vi "CircleShape.vi"(1 "Precision":i32, 2 "Y initial":dbl format="%#_13g", 3 "X initial":dbl format="%#_13g", 4 "Radius":dbl format="%#_13g") -> (0 "Output Point":dbl[][](array[numeric]))   [LabVIEW 2013]
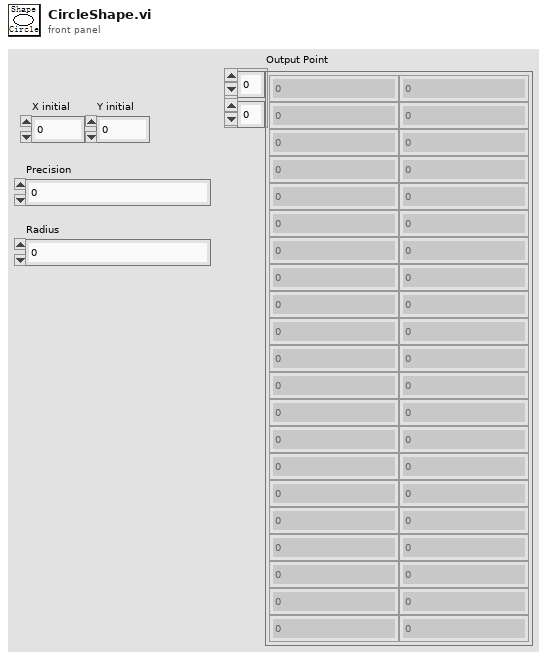
[diagram p1: front panel]
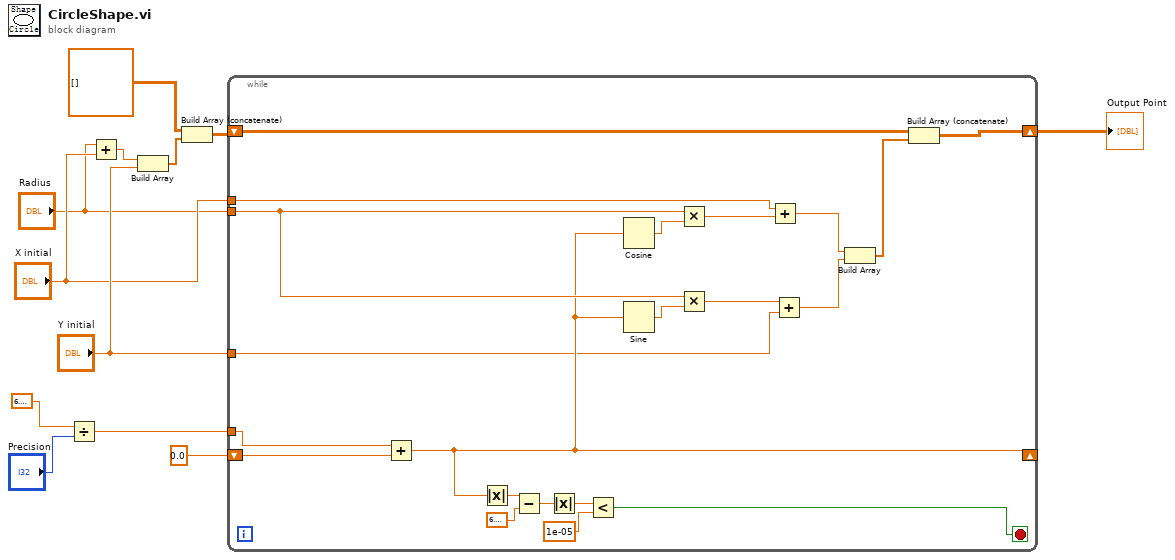
[diagram p0: block diagram]
diagram:
  n1 = Divide(x=6.283185307179586, y="Precision") -> (x/y=w9:dbl)
  n2 = Add(x="Radius", y="X initial") -> (x+y=w3:dbl)
  n3 = Build Array(w3, "Y initial") -> (w4:dbl[])
  n4 = Build Array (concatenate)(dbl[][] [], w4) -> (w6:dbl[][])
  n5 = while {
    tunnel: w9 -> [w32]
    shift-right: [w22] -> _
    shift-left: 0.0 -> [w33]
    tunnel: "Radius" -> [w23]
    shift-right: [w20] -> w8
    shift-left: w6 -> [w21]
    tunnel: "X initial" -> [w16]
    tunnel: "Y initial" -> [w15]
    stop <- w26 stop-if-true
    n6 = Add(x=w32, y=w33) -> (x+y=w22:dbl)
    n7 = Absolute Value(x=w22) -> (abs(x)=w31:dbl)
    n8 = Subtract(x=w31, y=6.283185307179586) -> (x-y=w29:dbl)
    n9 = Absolute Value(x=w29) -> (abs(x)=w28:dbl)
    n10 = Less?(x=w28, y=1e-05) -> (x < y?=w26:bool)
    n11 = Cosine(x=w22) -> (cos(x)=w24:dbl)
    n12 = Sine(x=w22) -> (sin(x)=w25:dbl)
    n13 = Multiply(x=w23, y=w24) -> (x*y=w18:dbl)
    n14 = Multiply(x=w23, y=w25) -> (x*y=w17:dbl)
    n15 = Add(x=w16, y=w18) -> (x+y=w14:dbl)
    n16 = Add(x=w17, y=w15) -> (x+y=w13:dbl)
    n17 = Build Array(w14, w13) -> (w19:dbl[])
    n18 = Build Array (concatenate)(w21, w19) -> (w20:dbl[][])
  }
  "Output Point" <- w8
